vi "setpoints.vi"() -> ()   [LabVIEW 2013]
uses:
  <vilib>/Utility/file.llb/Read From Spreadsheet File (DBL).vi
  Robot Global Data.vi
panel:
  in  "Default File":i32
  out "Number of Auton Files":i64
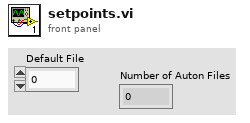
[diagram p1: front panel]
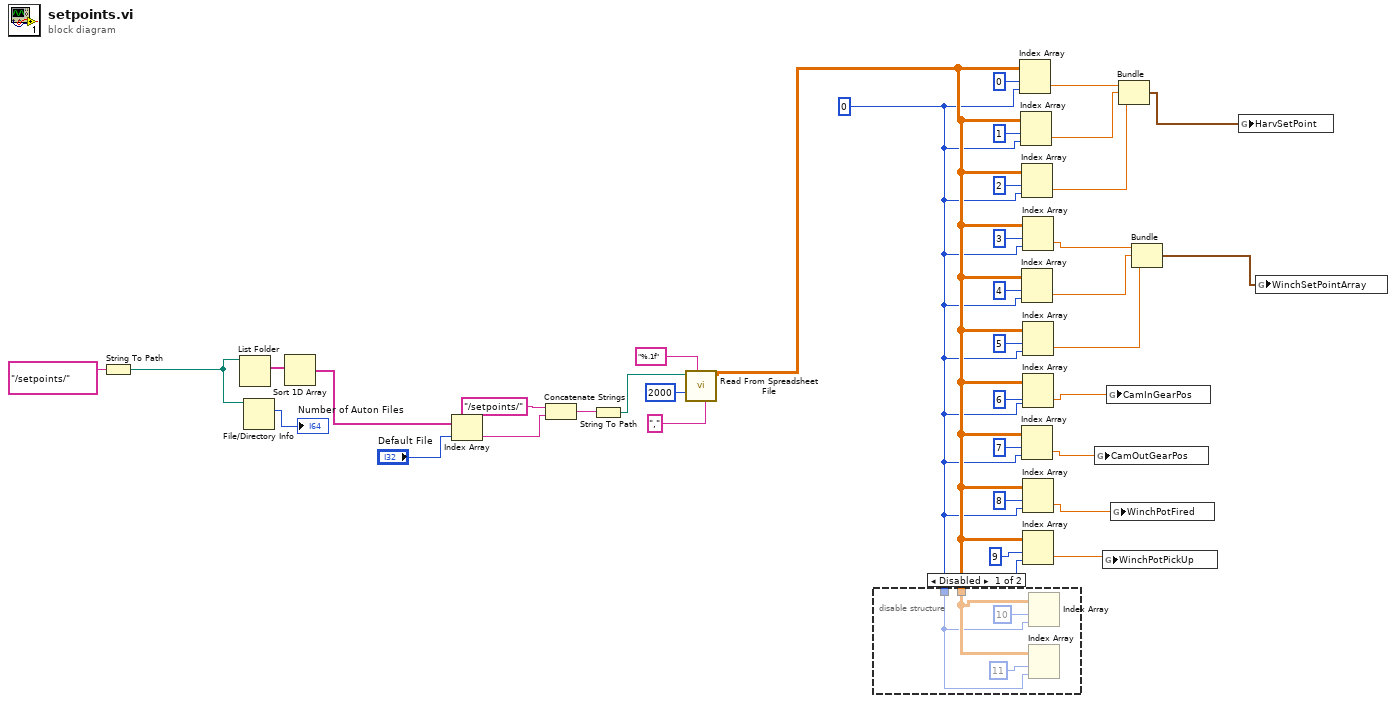
[diagram p0: block diagram]
diagram:
  w5 = 0
  n1 = String To Path(string="/setpoints/") -> (path=w28:path)
  n2 = List Folder(path=w28) -> (filenames=w29:string[])  [unwired: 1 in, 5 out]
  n3 = File/Directory Info(path=w28) -> (size=→"Number of Auton Files":i64)  [unwired: 1 in, 6 out]
  n4 = Sort 1D Array(array=w29) -> (sorted array=w31:string[])
  n5 = Index Array(array=w31, index="Default File") -> (element=w26:string)
  n6 = Concatenate Strings("/setpoints/" ("string"), w26) -> (w34:string)
  n7 = String To Path(string=w34) -> (path=w33:path)
  n8 = call-poly <vilib>:"Read From Spreadsheet File.vi"("delimiter (\\t)"="," ("delimiter (\\t)"), "format (%.3f)"="%.1f", "number of rows (all:-1)"=2000, "file path (dialog if empty)"=w33) -> ("all rows"=w6:dbl[][])  [unwired: 1 in, 6 out]
  n9 = disable-structure shown="Disabled" {
    disable-tunnel: w6 -> [w41 _]
    disable-tunnel: w5 -> [w40 _]
    frame Disabled {
      n10 = Index Array(array=w41, index (row)=10, index (col)=w40) -> ()  [unwired: 1 out]
      n11 = Index Array(array=w41, index (row)=11, index (col)=w40) -> ()  [unwired: 1 out]
    }
    frame Enabled {
    }
  }
  n12 = Index Array(array=w6, index (row)=0, index (col)=w5) -> (element=w16:dbl)
  n13 = Index Array(array=w6, index (row)=1, index (col)=w5) -> (element=w15:dbl)
  n14 = Index Array(array=w6, index (row)=2, index (col)=w5) -> (element=w14:dbl)
  n15 = Index Array(array=w6, index (row)=4, index (col)=w5) -> (element=w11:dbl)
  n16 = Index Array(array=w6, index (row)=7, index (col)=w5) -> (element=w8:dbl)
  n17 = Index Array(array=w6, index (row)=3, index (col)=w5) -> (element=w12:dbl)
  n18 = Index Array(array=w6, index (row)=5, index (col)=w5) -> (element=w10:dbl)
  n19 = Index Array(array=w6, index (row)=6, index (col)=w5) -> (element=w7:dbl)
  n20 = Index Array(array=w6, index (row)=8, index (col)=w5) -> (element=w3:dbl)
  n21 = Index Array(array=w6, index (row)=9, index (col)=w5) -> (element=w1:dbl)
  n22 = global write "Robot Global Data.vi" "CamOutGearPos"(w8) -> ()
  n23 = global write "Robot Global Data.vi" "WinchPotPickUp"(w1) -> ()
  n24 = global write "Robot Global Data.vi" "CamInGearPos"(w7) -> ()
  n25 = global write "Robot Global Data.vi" "WinchPotFired"(w3) -> ()
  n26 = Bundle(w16, w15, w14) -> (w13:cluster{dbl, dbl, dbl})  [unwired: 1 in]
  n27 = Bundle(w12, w11, w10) -> (w9:cluster{dbl, dbl, dbl})  [unwired: 1 in]
  n28 = global write "Robot Global Data.vi" "HarvSetPoint"(w13) -> ()
  n29 = global write "Robot Global Data.vi" "WinchSetPointArray"(w9) -> ()
